vi "Count Only Once Vr2.vi"(1 "InValue":bool, 2 "Action":enum16{"onPress", "onRelease", "Both"}(ring)) -> (0 "Result":bool)   [LabVIEW 2016]
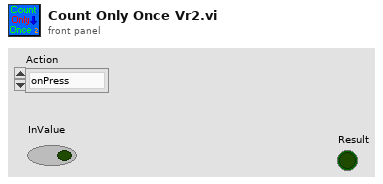
[diagram p1: front panel]
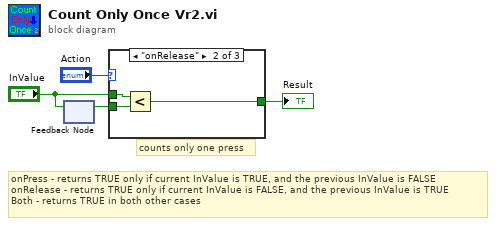
[diagram p0: block diagram]
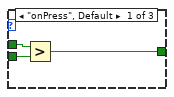
[diagram p2: hidden frame]
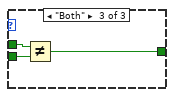
[diagram p3: hidden frame]
diagram:
  # "onPress - returns TRUE only if current InValue is TRUE, and the previous InValue is FALSE\nonRelease - returns TRUE only if current InValue is FALSE, and the previous InValue is TRUE\nBoth - returns TRUE in both other cases"
  # "counts only one press"
  n1 = feedback #1() -> (w3:bool)  [unwired: 1 in]
  n2 = feedback-in #1("InValue") -> ()
  n3 = case shown="\"onRelease\"" "Action" {
    tunnel: "InValue" -> [w7 w10 w13]
    tunnel: w3 -> [w6 w9 w12]
    tunnel: [w5 w8 w11] -> w1
    frame "onPress", Default {
      n4 = Greater?(x=w7, y=w6) -> (0:w5:bool)
    }
    frame "onRelease" {
      n5 = Less?(x=w10, y=w9) -> (x < y?=w8:bool)
    }
    frame "Both" {
      n6 = Not Equal?(x=w13, y=w12) -> (x != y?=w11:bool)
    }
  }
  "Result" <- w1
